vi "Draw matches in inspection image.vi"(10 "Raw matches":T2(array[cluster]), 11 "Image in":T1) -> (3 "Image out":T1)   [LabVIEW 2011]
uses:
  <vilib>/vision/Image Controls.llb/IMAQ Image.ctl
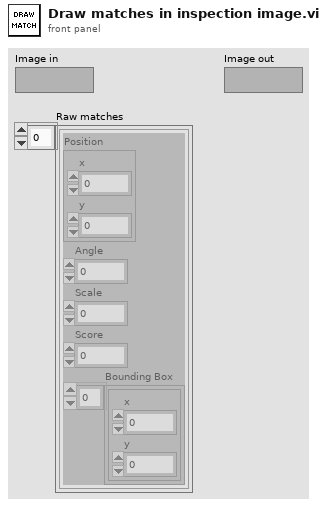
[diagram p1: front panel]
types:
  T1 = typedef "IMAQ Image.ctl" = refnum<image>
  T2 = cluster{"Position":cluster{"x":sgl, "y":sgl}, "Angle":sgl, "Scale":sgl, "Score":sgl, "Bounding Box":cluster{"x":sgl, "y":sgl}[]}[]
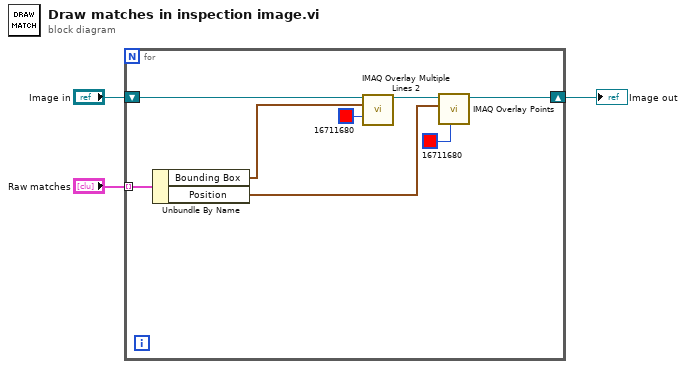
[diagram p0: block diagram]
diagram:
  n1 = for {
    shift-right: [w6] -> w2
    shift-left: "Image in" -> [w10]
    tunnel: "Raw matches" -> [w11] mode=indexing
    n2 = Unbundle By Name(w11) -> ("Bounding Box"=w9:cluster{"x":sgl, "y":sgl}[], "Position"=w5:cluster{"x":sgl, "y":sgl})
    n3 = call "IMAQ Overlay Multiple Lines 2"("Image"=w10, "Line End Points"=w9, "Color"=u32 16711680) -> ("Image Out"=w7:T1)  [unwired: 11 in, 1 out]
    n4 = call "IMAQ Overlay Points"("Color"=u32 16711680, "Point"=w5, "Image"=w7) -> ("Image Out"=w6:T1)  [unwired: 7 in, 1 out]
  }
  "Image out" <- w2
